vi "c ctre phoenixpro Request Control Follower.vi"(5 "OpposeMasterDirection":bool, 6 "MasterID":i32, 7 "cancelOtherRequests":bool, 8 "error in (no error)":errorcluster, 9 "updateTime":dbl, 10 "ecuEncoding":u32, 11 "canbus":string) -> (0 "error out":errorcluster, 3 "function return":i32)   [LabVIEW 2020, in "CTRE_PhoenixTools.lvlib"]
doc: "CTREXPORT int c_ctre_phoenixpro_RequestControlFollower(const char *canbus, uint32_t ecuEncoding, double updateTime, bool cancelOtherRequests, int MasterID, bool OpposeMasterDirection);"
uses:
  CTRE_PhoenixTools.lvlib
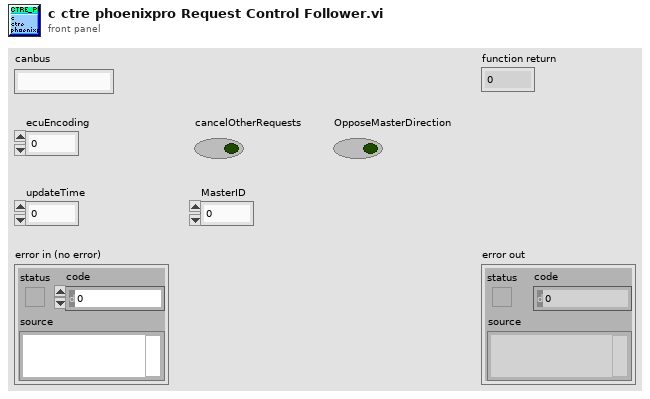
[diagram p1: front panel]
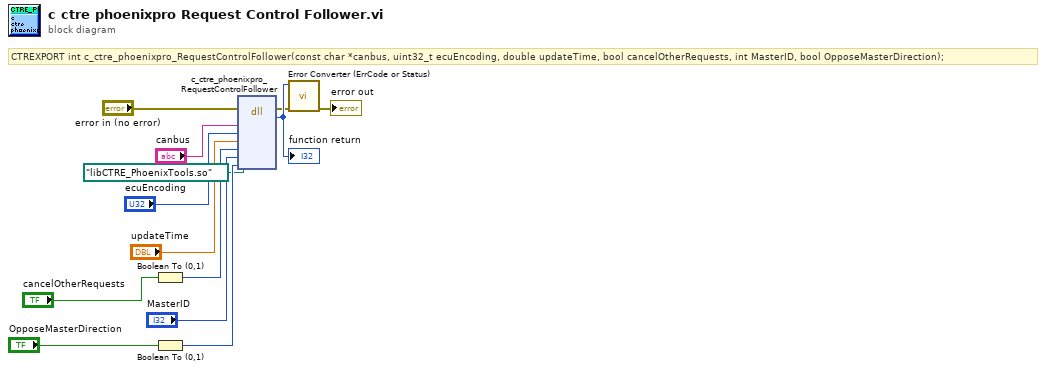
[diagram p0: block diagram]
diagram:
  # "CTREXPORT int c_ctre_phoenixpro_RequestControlFollower(const char *canbus, uint32_t ecuEncoding, double updateTime, bool cancelOtherRequests, int MasterID, bool OpposeMasterDirection);"
  n1 = Boolean To (0,1)(Boolean="cancelOtherRequests") -> (0, 1=w8:i16)
  n2 = Boolean To (0,1)(Boolean="OpposeMasterDirection") -> (0, 1=w5:i16)
  n3 = dll-call lib="?" fn="c_ctre_phoenixpro_RequestControlFollower"(path in=path "libCTRE_PhoenixTools.so", error in="error in (no error)", "canbus"="canbus", "ecuEncoding"="ecuEncoding", "updateTime"="updateTime", "cancelOtherRequests"=w8, "MasterID"="MasterID", "OpposeMasterDirection"=w5) -> (error out=w3:errorcluster, w13:i32)  [unwired: 7 in, 1 out]
  "function return" <- w13
  n4 = call "Error Converter (ErrCode or Status).vi"("error in (no error)"=w3, "error code"=w13) -> ("error out"=→"error out":errorcluster)  [unwired: 9 in]
